vi "GEOM_CorrYcoord_dataonly.vi"(10 "levels":cluster{"amplifiers":i32, "coord":i32}[](array[cluster]), 11 "Array":T1[](array[typedef]) {"fliped" items=["none", "horizontal", "vertical"]; "type" items=["LL", "LR", "UL", "UR"]}) -> (1 "ycoord":u32, 3 "Array 2":T1[](array[typedef]) {"fliped" items=["none", "horizontal", "vertical"]; "type" items=["LL", "LR", "UL", "UR"]})   [LabVIEW 2016]
uses:
  GEOM_Amplifier.ctl
  GEOM_AmpType.ctl
  GEOM_ROI.ctl
  GEOM_Coords.ctl
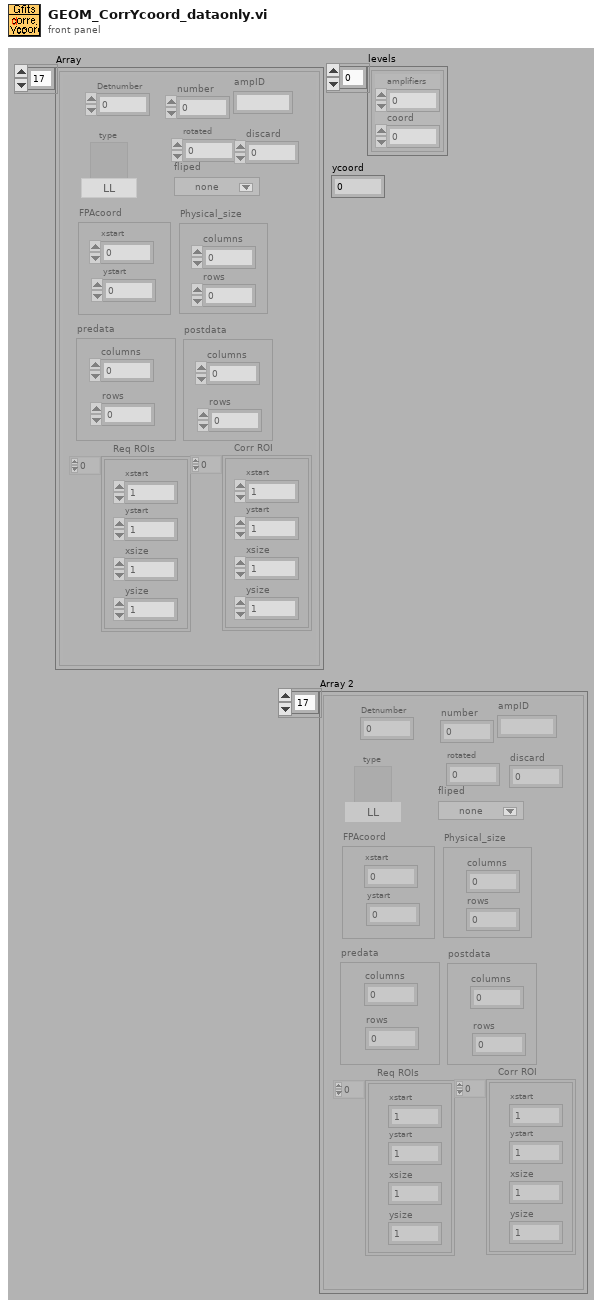
[diagram p1: front panel]
types:
  T1 = typedef "GEOM_Amplifier.ctl" = cluster{"number":i32, "type":T2, "rotated":i16, "fliped":u16, "FPAcoord":cluster{"xstart":i32, "ystart":i32}, "Physical_size":cluster{"columns":i32, "rows":i32}, "predata":cluster{"columns":i32, "rows":i32}, "postdata":cluster{"columns":i32, "rows":i32}, "Req ROIs":T3, "Corr ROI":T3, "Detnumber":i32, "ampID":string, "discard":i32}
  T2 = typedef "GEOM_AmpType.ctl" = u16
  T3 = typedef "GEOM_ROI.ctl" = T4[]
  T4 = typedef "GEOM_Coords.ctl" = cluster{"xstart":u32, "ystart":u32, "xsize":u32, "ysize":u32}
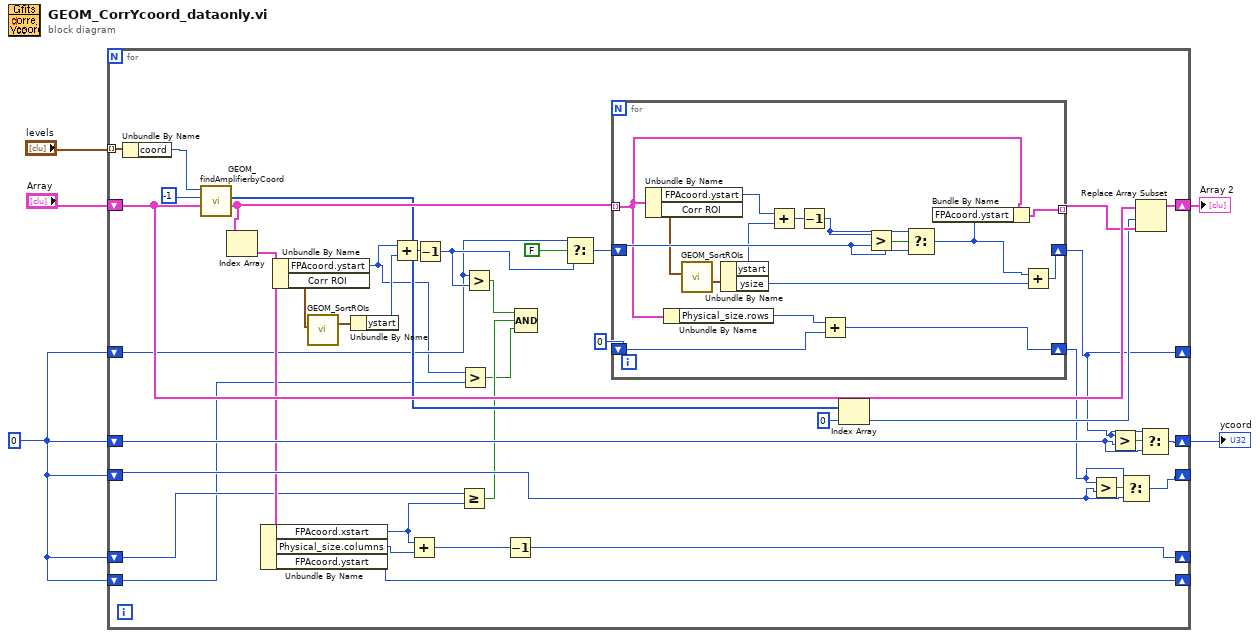
[diagram p0: block diagram]
diagram:
  w1 = u32 0
  n1 = for {
    tunnel: "levels" -> [w44] mode=indexing
    shift-right: [w39] -> w4
    shift-left: "Array" -> [w43]
    shift-right: [w38] -> w3
    shift-left: w1 -> [w36]
    shift-right: [w28] -> _
    shift-left: w1 -> [w29]
    shift-right: [w7] -> _
    shift-left: w1 -> [w20]
    shift-right: [w15] -> _
    shift-left: w1 -> [w14]
    shift-right: [w13] -> _
    shift-left: w1 -> [w10]
    n2 = Unbundle By Name(w44) -> ("coord"=w8:i32)
    n3 = call "GEOM_findAmplifierbyCoord.vi"("amplifiers"=w43, "ycoord"=-1 ("xcoord"), "xcoord"=w8) -> ("amplifiers"=w32:T1[], "indexes"=w27:i32[])  [unwired: 7 out]
    n4 = Index Array(array=w32) -> (element=w24:T1)  [unwired: 1 in]
    n5 = Unbundle By Name(w24) -> ("FPAcoord.xstart"=w18:i32, "Physical_size.columns"=w23:i32, "FPAcoord.ystart"=w13:i32)
    n6 = Unbundle By Name(w24) -> ("FPAcoord.ystart"=w11:i32, "Corr ROI"=w35:T3)
    n7 = call "GEOM_SortROIs.vi"("ROIs"=w35) -> ("Extreme Coords"=w34:T4)  [unwired: 10 out]
    n8 = Unbundle By Name(w34) -> ("ystart"=w25:u32)
    n9 = Add(x=w11, y=w25) -> (x+y=w33:u32)
    n10 = Add(x=w18, y=w23) -> (x+y=w19:i32)
    n11 = Decrement(x=w33) -> (x-1=w16:u32)
    n12 = Greater Or Equal?(x=w20, y=w18) -> (x >= y?=w22:bool)
    n13 = Greater?(x=w11, y=w10) -> (0:w12:bool)
    n14 = Greater?(x=w14, y=w16) -> (0:w21:bool)
    n15 = Decrement(x=w19) -> (x-1=w7:i32)
    n16 = Compound Arithmetic op=AND(w21, w22, w12) -> ()  [unwired: 1 out]
    n17 = Select(t=w14, s=FALSE, f=w16) -> (s? t:f=w17:u32)
    n18 = for {
      tunnel: w32 -> [w51] mode=indexing
      shift-right: [w58] -> w15
      shift-left: w17 -> [w59]
      tunnel: [w60] -> w42 mode=indexing
      shift-right: [w48] -> w30
      shift-left: 0 -> [w49]
      n19 = Unbundle By Name(w51) -> ("FPAcoord.ystart"=w53:i32, "Corr ROI"=w57:T3)
      n20 = Unbundle By Name(w51) -> ("Physical_size.rows"=w50:i32)
      n21 = call "GEOM_SortROIs.vi"("ROIs"=w57) -> ("Extreme Coords"=w56:T4)  [unwired: 10 out]
      n22 = Unbundle By Name(w56) -> ("ystart"=w55:u32, "ysize"=w47:u32)
      n23 = Add(x=w53, y=w55) -> (x+y=w54:u32)
      n24 = Decrement(x=w54) -> (x-1=w52:u32)
      n25 = Add(x=w50, y=w49) -> (x+y=w48:i32)
      n26 = Greater?(x=w52, y=w59) -> (0:w46:bool)
      n27 = Select(t=w52, s=w46, f=w59) -> (s? t:f=w45:u32)
      n28 = Bundle By Name(cluster=w51, "FPAcoord.ystart"=w45) -> (w60:T1)
      n29 = Add(x=w45, y=w47) -> (x+y=w58:u32)
    }
    n30 = Index Array(array=w27, index=0) -> (element=w40:i32)
    n31 = Greater?(x=w30, y=w29) -> (0:w31:bool)
    n32 = Greater?(x=w15, y=w36) -> (0:w37:bool)
    n33 = Select(t=w30, s=w31, f=w29) -> (s? t:f=w28:u32)
    n34 = Replace Array Subset(array=w43, new element=w42, index=w40) -> (w39:T1[])
    n35 = Select(t=w15, s=w37, f=w36) -> (s? t:f=w38:u32)
  }
  "Array 2" <- w4
  "ycoord" <- w3
